vi "gain.vi"() -> ()   [LabVIEW 2009]
uses:
  <vilib>/imath/engines/lvmath2/RunTimeEngine/ErrorHandling/NIMS_Finalize Error.vi
  <vilib>/imath/engines/lvmath2/RunTimeEngine/Parser/MC_Version.vi
  <vilib>/imath/engines/lvmath2/RunTimeEngine/Managers/WorkSpace/UID Generator.vi
  <vilib>/imath/engines/lvmath2/RunTimeEngine/NodeEndStatement/NIMS_NodeEndStatement_Output.vi
  <instcachedir>/0/NIMS_NodeEndStatement_Output_B70DDD75627E4997AAE11E9955EDAA25.lvgen/NIMS_NodeEndStatement_Output_B70DDD75627E4997AAE11E9955EDAA25_001.vi
  <vilib>/imath/engines/lvmath2/RunTimeEngine/Managers/SymbolTable/Clear UID.vi
  <vilib>/imath/engines/lvmath/Functions/Error Handling/MergeErrorsWrapper.vi
  <vilib>/imath/engines/lvmath2/RunTimeEngine/LocalVariableDefStatement/MC_LocalVariableDefStatement_Display.vi
  <vilib>/imath/engines/lvmath2/RunTimeEngine/RunTimeType/NIMS_RunTimeType_From StrictType (excl LVString).vi
  <vilib>/imathl/engines/lvmath/Functions/Error Handling/Create Error.vi
  <vilib>/imath/engines/lvmath2/RunTimeEngine/VariableToken/Read/NIMS_Get Elements - RV(_) - Check.vi
  <instcachedir>/0/NIMS_Get Elements - RV(_) - Check_60F12861D0564803969A5D0D0D1716CD.lvgen/NIMS_Get Elements - RV(_) - Check_60F12861D0564803969A5D0D0D1716CD_000.vi
  <instcachedir>/0/NIMS_NodeEndStatement_Output_B70DDD75627E4997AAE11E9955EDAA25.lvgen/NIMS_NodeEndStatement_Output_B70DDD75627E4997AAE11E9955EDAA25_000.vi
  <vilib>/imath/engines/lvmath2/RunTimeEngine/RangeToken/NIMS_Range.vi
  <instcachedir>/0/NIMS_Range_6D647EC16A744C98B5DE1D649A2D648D.lvgen/NIMS_Range_6D647EC16A744C98B5DE1D649A2D648D_001.vi
  <vilib>/imath/engines/lvmath/Functions/Error Handling/error.ctl
  <vilib>/imath/engines/lvmath2/RunTimeEngine/VariableToken/NIMS_VariableToken_CondDefined.vi
  <instcachedir>/0/NIMS_VariableToken_CondDefined_5641E79000FB4D628475532441475385.lvgen/NIMS_VariableToken_CondDefined_5641E79000FB4D628475532441475385_001.vi
  <vilib>/imath/engines/lvmath/Functions/Error Handling/MC_Mask_Errors.vi
  <vilib>/imath/engines/lvmath2/RunTimeEngine/BuiltInFunctions/rem/NIMS_rem_no checks.vi
  <instcachedir>/0/NIMS_rem_no checks_4CC9B305AB7E42EF90AFC4973FB32F8D.lvgen/NIMS_rem_no checks_4CC9B305AB7E42EF90AFC4973FB32F8D_000.vi
  <vilib>/imath/engines/lvmath2/RunTimeEngine/BuiltInFunctions/uint32/NIMS_uint32(real).vi
  <instcachedir>/0/NIMS_uint32(real)_FDC83D68D45943DDB8F3F934FF8A712F.lvgen/NIMS_uint32(real)_FDC83D68D45943DDB8F3F934FF8A712F_000.vi
  <vilib>/imath/engines/lvmath2/RunTimeEngine/BuiltInFunctions/double/NIMS_double.vi
  <instcachedir>/0/NIMS_double_2CE444F3CE4146B199A482FE12545E45.lvgen/NIMS_double_2CE444F3CE4146B199A482FE12545E45_000.vi
  <vilib>/imath/engines/lvmath2/RunTimeEngine/BuiltInFunctions/length/NIMS_length(GV).vi
  <instcachedir>/0/NIMS_length(GV)_7D6E94E728E145E68721C53861296D96.lvgen/NIMS_length(GV)_7D6E94E728E145E68721C53861296D96_000.vi
  <instcachedir>/0/NIMS_Range_6D647EC16A744C98B5DE1D649A2D648D.lvgen/NIMS_Range_6D647EC16A744C98B5DE1D649A2D648D_000.vi
  <vilib>/imath/engines/lvmath2/RunTimeEngine/ReplaceToken/NIMS_Replace - V(S)=S.vi
  <instcachedir>/0/NIMS_Replace - V(S)=S_670A9E0533664C1D848C8E58B3321B6A.lvgen/NIMS_Replace - V(S)=S_670A9E0533664C1D848C8E58B3321B6A_002.vi
  <vilib>/imath/engines/lvmath2/RunTimeEngine/ReplaceToken/NIMS_Replace - Size Check _(_)=S.vi
  <instcachedir>/0/NIMS_Replace - Size Check _(_)=S_8596181D73404097BAB9CBB006194BB0.lvgen/NIMS_Replace - Size Check _(_)=S_8596181D73404097BAB9CBB006194BB0_002.vi
  <vilib>/imath/engines/lvmath2/RunTimeEngine/ReplaceToken/NIMS_Replace - Check Linear.vi
  <instcachedir>/0/NIMS_Replace - Check Linear_9243CBB174894FF6977027453DA6955E.lvgen/NIMS_Replace - Check Linear_9243CBB174894FF6977027453DA6955E_002.vi
  <vilib>/imath/engines/lvmath2/RunTimeEngine/VariableToken/NIMS_VariableToken_CondDefinedDefinedByReplace.vi
  <instcachedir>/0/NIMS_VariableToken_CondDefinedDefinedByReplace_D162CFFC24174562A9FEA619A91E1A56.lvgen/NIMS_VariableToken_CondDefinedDefinedByReplace_D162CFFC24174562A9FEA619A91E1A56_002.vi
  <vilib>/imath/engines/lvmath2/RunTimeEngine/CommandStatement/MC_CommandStatement_break.vi
  <vilib>/imath/engines/lvmath2/RunTimeEngine/ArithmeticOperatorToken/NIMS_ArithmeticOperator_times.vi
  <instcachedir>/0/NIMS_ArithmeticOperator_times_3987BC660D7947CD8628C10658A43225.lvgen/NIMS_ArithmeticOperator_times_3987BC660D7947CD8628C10658A43225_001.vi
  <instcachedir>/0/NIMS_ArithmeticOperator_times_3987BC660D7947CD8628C10658A43225.lvgen/NIMS_ArithmeticOperator_times_3987BC660D7947CD8628C10658A43225_000.vi
  <vilib>/imath/engines/lvmath2/RunTimeEngine/Managers/SymbolTable/NIMS_WorkSpace.lvlib
panel:
  in  "?":enum32{"GAIN MEASUREMENT"}(tab)
  out "XY Graph 2":cluster{"Y":dbl[], "Y":dbl[]}[](graph)
  in  "Samples":i32=3 min=3 max=50 step=1
  out "G":dbl
  out "m":dbl
  in  "?":enum32{"ATTENUATOR"}(tab)
  out "?":dbl[](graph)
  in  "Set the value of attenuation in dB":dbl(slide) scale=0.0..100.0
  out "?":errorcluster
  in  "HELP FOR ATTENUATOR":bool
  out "error out":errorcluster
  in  "?":enum32{"ISOLATOR"}(tab)
  out "?":dbl[](graph)
  in  "?":bool
  out "?":errorcluster
  in  "HELP FOR ISOLATOR":bool
  out "error out":errorcluster
  in  "?":enum32{"MODULATOR"}(tab)
  in  "Modulating Frequency(KHz)":dbl(slide) scale=0.5..1.5
  out "?":errorcluster
  out "?":dbl[](graph)
  in  "HELP FOR MODULATOR":bool
  out "error out":errorcluster
  in  "?":enum32{"SOURCE"}(tab)
  out "?":dbl[](graph)
  in  "Frequency of carrier wave(GHz)":dbl(slide) scale=8.0..15.0
  in  "Voltage":dbl(knob) scale=0.0..20.0 scale format="%#_10g"
  out "?":errorcluster
  in  "HELP FOR SOURCE":bool
  out "error out":errorcluster
  # "Source"
  # "Attenuator"
  # "VSWR meter"
  # "Coaxial to rectangular adapter"
  # "Transmitting and Recieving Antenna"
  # "Connecting Waveguide"
  # "Connecting Waveguide"
  # "Isolator"
  # "Formula Used"
  # "Backward Direction"
  # "Forward direction"
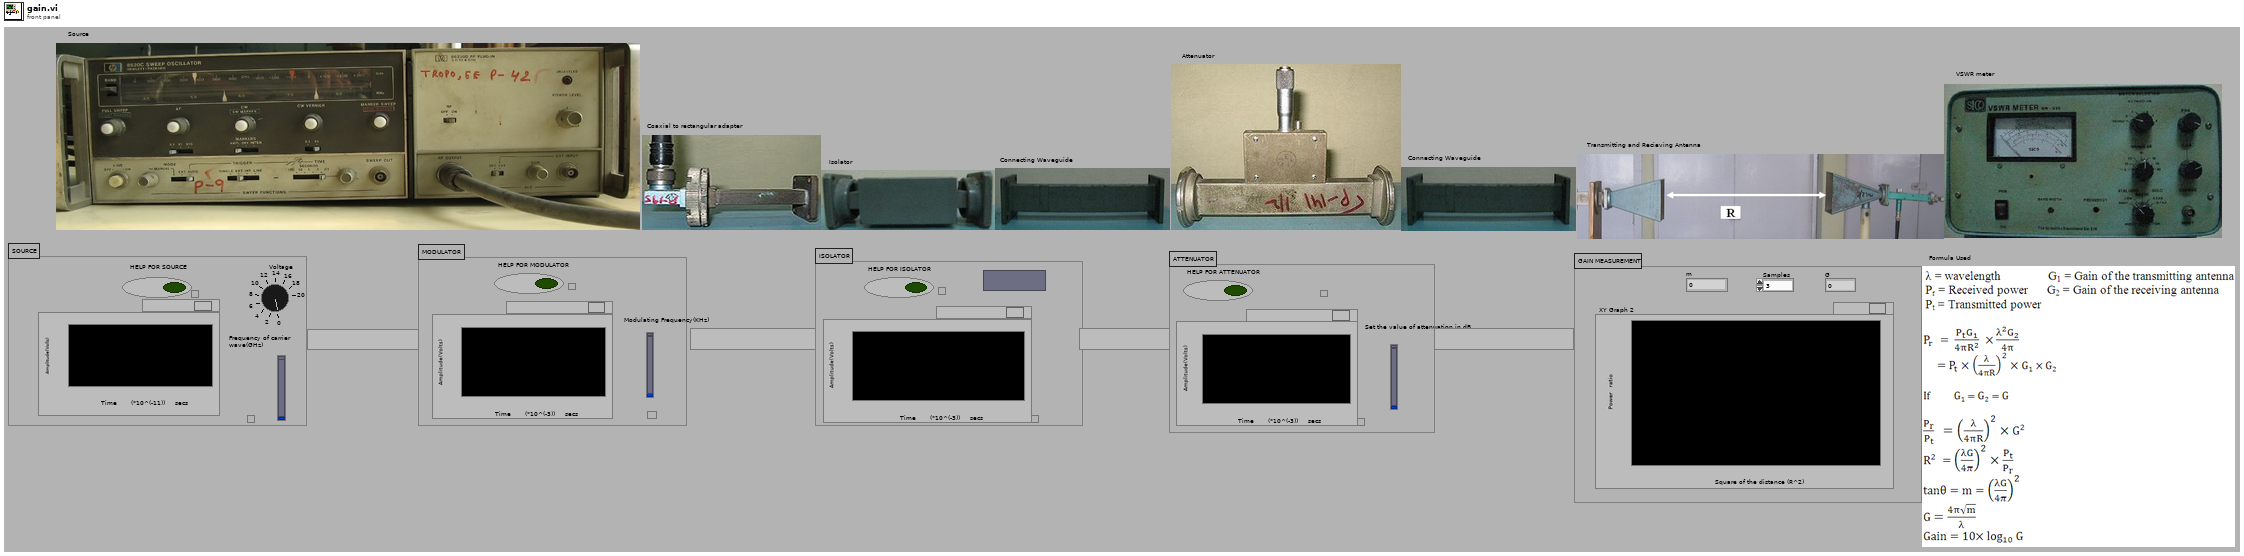
[diagram p1: front panel]
types:
  T1 = typedef "imagedata.ctl" = cluster{"image type":i32, "image depth":i32, "image":u8[], "mask":u8[], "colors":u32[], "Rectangle":cluster{"left":i16, "top":i16, "right":i16, "bottom":i16}}
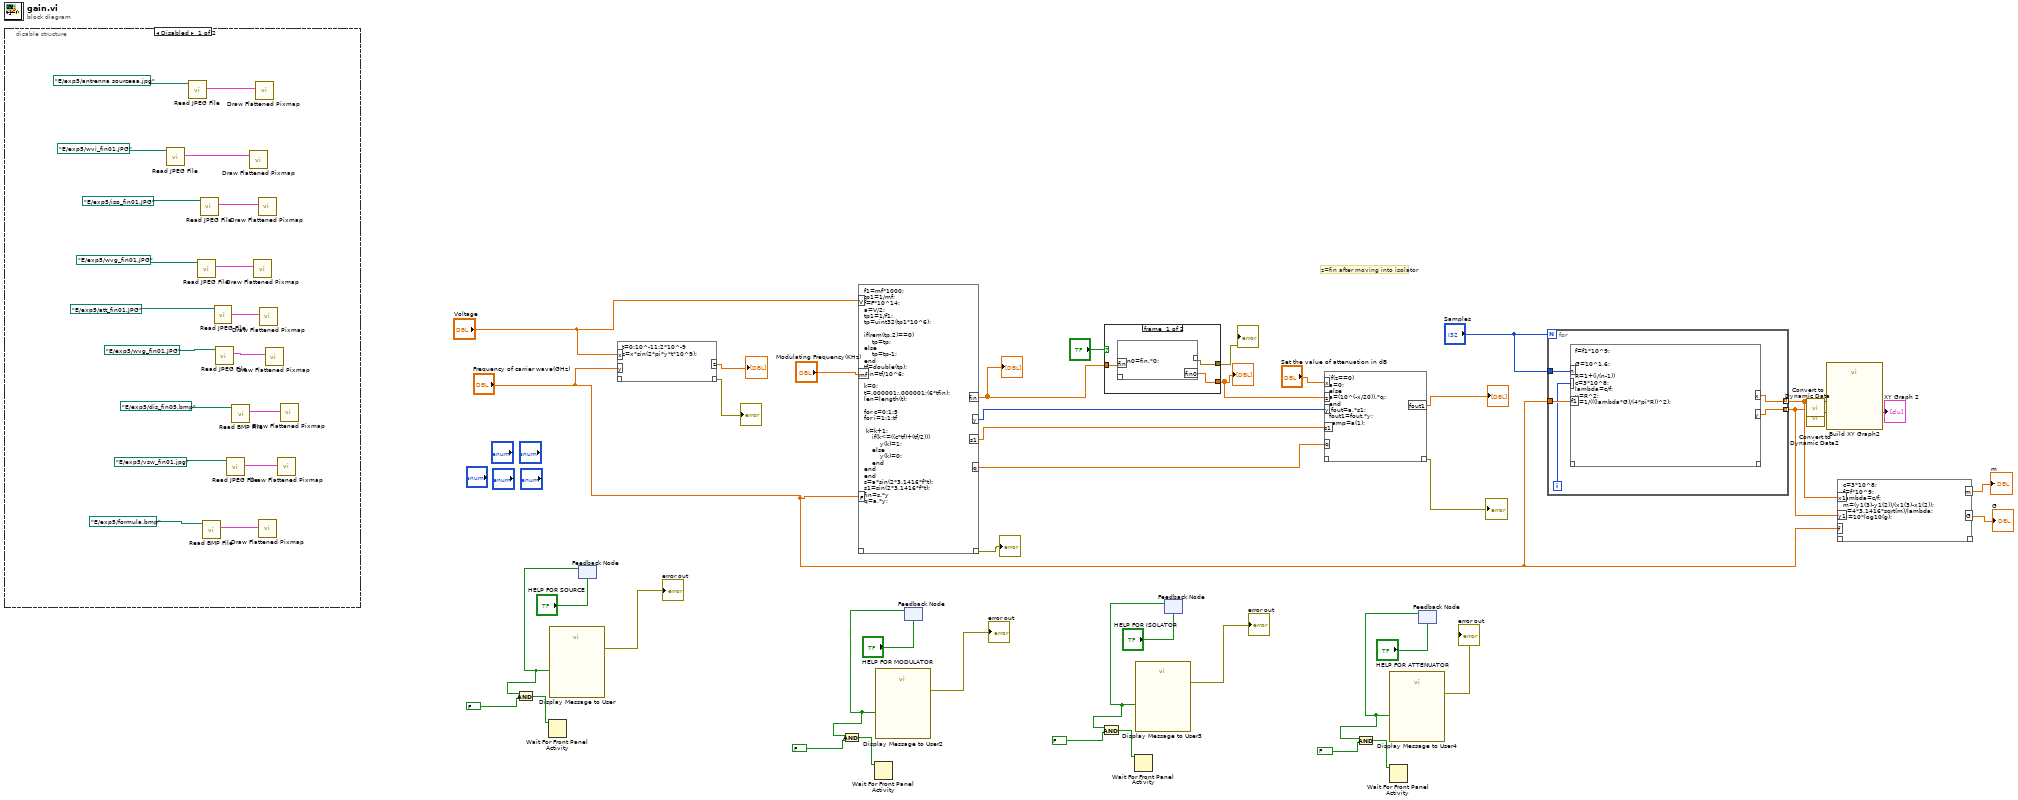
[diagram p0: block diagram]
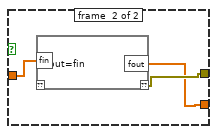
[diagram p3: hidden frame]
diagram:
  # "z=fin after moving into isolator"
  n1 = disable-structure shown="Disabled" {
    frame #0 {
      n2 = call <vilib>:"Read JPEG File.vi"("path to JPEG file"=path "E:/exp5/wvi_fin01.JPG" ("coaxial rectangular adapter")) -> ("image data"=w66:T1)  [unwired: 8 in, 2 out]
      n3 = call <vilib>:"Read JPEG File.vi"("path to JPEG file"=path "E:/exp5/antrenna sourceaa.jpg" ("Source")) -> ("image data"=w56:T1)  [unwired: 8 in, 2 out]
      n4 = call <vilib>:"Read JPEG File.vi"("path to JPEG file"=path "E:/exp5/wvg_fin01.JPG" ("Connecting waveguide")) -> ("image data"=w51:T1)  [unwired: 8 in, 2 out]
      n5 = call <vilib>:"Read JPEG File.vi"("path to JPEG file"=path "E:/exp5/iso_fin01.JPG" ("Isolator")) -> ("image data"=w54:T1)  [unwired: 8 in, 2 out]
      n6 = call <vilib>:"Read BMP File.vi"("path to BMP file"=path "E:/exp5/formula.bmp" ("formula")) -> ("image data"=w50:T1)  [unwired: 8 in, 2 out]
      n7 = call <vilib>:"Read JPEG File.vi"("path to JPEG file"=path "E:/exp5/att_fin01.JPG" ("Variable Attenuator 2")) -> ("image data"=w62:T1)  [unwired: 8 in, 2 out]
      n8 = call <vilib>:"Read JPEG File.vi"("path to JPEG file"=path "E:/exp5/wvg_fin01.JPG" ("Connecting Waveguide 2")) -> ("image data"=w64:T1)  [unwired: 8 in, 2 out]
      n9 = call <vilib>:"Read JPEG File.vi"("path to JPEG file"=path "E:/exp5/vsw_fin01.jpg" ("VSWR meter 2")) -> ("image data"=w60:T1)  [unwired: 8 in, 2 out]
      n10 = call <vilib>:"Read BMP File.vi"("path to BMP file"=path "E:/exp5/dis_fin05.bmp" ("Tx and Rx")) -> ("image data"=w59:T1)  [unwired: 8 in, 2 out]
      n11 = call <vilib>:"Draw Flattened Pixmap.vi"("image data"=w66) -> ()  [unwired: 8 in, 1 out]
      n12 = call <vilib>:"Draw Flattened Pixmap.vi"("image data"=w51) -> ()  [unwired: 8 in, 1 out]
      n13 = call <vilib>:"Draw Flattened Pixmap.vi"("image data"=w56) -> ()  [unwired: 8 in, 1 out]
      n14 = call <vilib>:"Draw Flattened Pixmap.vi"("image data"=w54) -> ()  [unwired: 8 in, 1 out]
      n15 = call <vilib>:"Draw Flattened Pixmap.vi"("image data"=w50) -> ()  [unwired: 8 in, 1 out]
      n16 = call <vilib>:"Draw Flattened Pixmap.vi"("image data"=w62) -> ()  [unwired: 8 in, 1 out]
      n17 = call <vilib>:"Draw Flattened Pixmap.vi"("image data"=w64) -> ()  [unwired: 8 in, 1 out]
      n18 = call <vilib>:"Draw Flattened Pixmap.vi"("image data"=w60) -> ()  [unwired: 8 in, 1 out]
      n19 = call <vilib>:"Draw Flattened Pixmap.vi"("image data"=w59) -> ()  [unwired: 8 in, 1 out]
    }
    frame #1 {
    }
  }
  n20 = feedback #1("HELP FOR SOURCE") -> (w43:bool)
  n21 = And(x=w43, y=FALSE) -> (x .and. y?=w41:bool)
  n22 = Wait For Front Panel Activity(3:w41) -> ()  [unwired: 3 out]
  n23 = call "Display Message to User"("Enable"=w43) -> ("error out"=→"error out":errorcluster, "CLOSE"=w45:bool)  [unwired: 2 in, 7 out]
  n24 = mathscript code="t=0:10^-11:2*10^-9\nz=x*sin(2*pi*y*t*10^9);"("x"="Voltage", "y"="Frequency of carrier wave(GHz)") -> ("??"=→"?":errorcluster, "z"=→"?":dbl[])  [unwired: 1 in]
  n25 = mathscript code="f1=mf*1000;\ntp1=1/mf;\nf=F*10^14;\na=V/2;\ntp1=1/f1;\ntp=uint32(tp1*10^6);\n\nif(rem(tp,2)==0)\n    tp=tp;\nelse\n    tp=tp-1;\nend\ntf=double(tp);\ntfin=tf/10^6;\n\nk=0;\nt=.000001:.000001:(6*tfin);\nlen=length(t);\n\nfor c=0:1:5\nfor i=1:1:tf\n  \n k=k+1;\n    if(k<=((c*tf)+(tf/2)))\n        y(k)=1;\n    else\n        y(k)=0;\n    end\nend\nend\ns=a*sin(2*3.1416*f*t);\ns1=sin(2*3.1416*f*t);\nfin=s.*y\nq=a.*y;"("V"="Voltage", "mf"="Modulating Frequency(KHz)", "F"="Frequency of carrier wave(GHz)") -> ("??"=→"?":errorcluster, "fin"=w2:dbl[], "y"=w6:i32[], "q"=w7:dbl[], "s1"=w5:dbl[])  [unwired: 1 in]
  "?" <- w2
  n26 = feedback #2("HELP FOR MODULATOR") -> (w37:bool)
  n27 = And(x=w37, y=FALSE) -> (x .and. y?=w35:bool)
  n28 = Wait For Front Panel Activity(3:w35) -> ()  [unwired: 3 out]
  n29 = call "Display Message to User2"("Enable"=w37) -> ("error out"=→"error out":errorcluster, "CLOSE"=w39:bool)  [unwired: 2 in, 7 out]
  n30 = case shown="True" "?" {
    tunnel: w2 -> [w67 w90]
    tunnel: [w69 w89] -> w47
    tunnel: [w68 w88] -> w3
    frame #0 {
      n31 = mathscript code="fin0=fin.*0;"("fin"=w67) -> ("??"=w69:errorcluster, "fin0"=w68:dbl[])  [unwired: 1 in]
    }
    frame #1 {
      n32 = mathscript code="fout=fin"("fin"=w90) -> ("??"=w89:errorcluster, "fout"=w88:dbl[])  [unwired: 1 in]
    }
  }
  "?" <- w3
  "?" <- w47
  n33 = feedback #3("HELP FOR ISOLATOR") -> (w31:bool)
  n34 = And(x=w31, y=FALSE) -> (x .and. y?=w29:bool)
  n35 = Wait For Front Panel Activity(3:w29) -> ()  [unwired: 3 out]
  n36 = call "Display Message to User3"("Enable"=w31) -> ("error out"=→"error out":errorcluster, "CLOSE"=w33:bool)  [unwired: 2 in, 7 out]
  n37 = mathscript code="if(z==0)\na=0;\nelse\na=(10^(-x/20)).*q;\nend\n fout=a.*s1;\nfout1=fout.*y;\nsamp=a(1);"("x"="Set the value of attenuation in dB", "z"=w3, "y"=w6, "s1"=w5, "q"=w7) -> ("??"=→"?":errorcluster, "fout1"=→"?":dbl[])  [unwired: 1 in]
  n38 = feedback #4("HELP FOR ATTENUATOR") -> (w25:bool)
  n39 = And(x=w25, y=FALSE) -> (x .and. y?=w23:bool)
  n40 = Wait For Front Panel Activity(3:w23) -> ()  [unwired: 3 out]
  n41 = call "Display Message to User4"("Enable"=w25) -> ("error out"=→"error out":errorcluster, "CLOSE"=w27:bool)  [unwired: 2 in, 7 out]
  n42 = for {
    N: "Samples" -> [_]
    tunnel: "Frequency of carrier wave(GHz)" -> [w127]
    tunnel: "Samples" -> [w126]
    tunnel: [w125] -> w18 mode=indexing
    tunnel: [w124] -> w15 mode=indexing
    i -> [w123]
    n43 = mathscript code="f=f1*10^9;\n\nG=10^1.6;\n\nR=1+(i/(n-1))\nc=3*10^8;\nlambda=c/f;\ny=R^2;\nx=1/(((lambda*G)/(4*pi*R))^2);"("f1"=w127, "n"=w126, "i"=w123) -> ("y"=w124:dbl, "x"=w125:dbl)  [unwired: 2 out]
  }
  n44 = call "Convert to Dynamic Data"("Array"=w18) -> ("Dynamic Data Type"=w21:dynamicdata)  [unwired: 3 out]
  n45 = call "Convert to Dynamic Data2"("Array"=w15) -> ("Dynamic Data Type"=w20:dynamicdata)  [unwired: 3 out]
  n46 = call "Build XY Graph2"("Y Input"=w20, "X Input"=w21) -> ("XY Graph"=→"XY Graph 2":cluster{"Y":dbl[], "Y":dbl[]}[])  [unwired: 3 in, 6 out]
  n47 = mathscript code="c=3*10^8;\nf=f*10^9;\nlambda=c/f;\nm=(y1(3)-y1(2))/(x1(3)-x1(2));\ng=4*3.1416*sqrt(m)/lambda;\nG=10*log10(g);"("x1"=w18, "y1"=w15, "f"="Frequency of carrier wave(GHz)") -> ("m"=→"m":dbl, "G"=→"G":dbl)  [unwired: 2 out]
